vi "plant_structure.vi"(9 "Dataflow":errorcluster, 10 "Pause":refnum<vi>, 11 "Stop":refnum<vi>) -> ()   [LabVIEW 2019]
uses:
  lib/libSimulationControl/libSimulationControl.lvlib
panel:
  out "Dataflow Out":errorcluster
  # "*******************************************************************\nBiogas Plant Control\n\nAuthor: Paul Zügel\nGCSC-Frankfurt am Main 2020\n\n*******************************************************************"
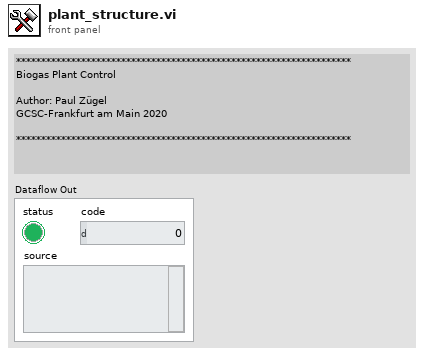
[diagram p1: front panel]
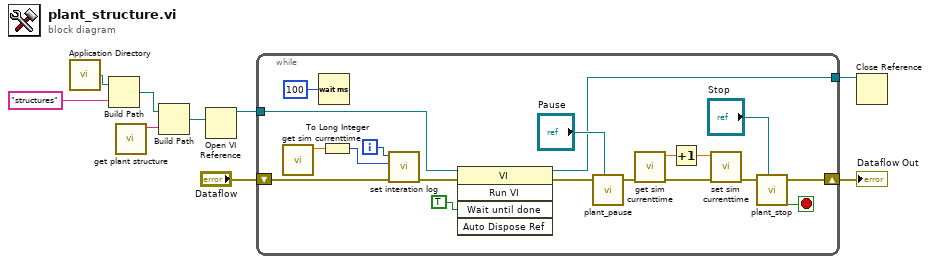
[diagram p0: block diagram]
diagram:
  n1 = call <vilib>:"Application Directory.vi"() -> ("Application Directory"=w7:path)
  n2 = Build Path(base path=w7, name or relative path="structures") -> (appended path=w5:path)
  n3 = call "get plant structure.vi"() -> ("function return"=w4:string)  [unwired: 10 in, 1 out]
  n4 = Build Path(base path=w5, name or relative path=w4) -> (appended path=w6:path)
  n5 = Open VI Reference(vi path=w6) -> (vi reference=w2:refnum<vi>)  [unwired: 5 in, 1 out]
  n6 = while {
    shift-right: [w25] -> w8
    shift-left: "Dataflow" -> [w15]
    tunnel: w2 -> [w13]
    tunnel: [w12] -> w1
    i -> [w24]
    stop <- w21 stop-if-true
    n7 = call "get sim currenttime.vi"() -> ("current_time"=w11:dbl)  [unwired: 10 in, 1 out]
    n8 = Wait (ms)(milliseconds to wait=u32 100) -> ()  [unwired: 1 out]
    n9 = To Long Integer(number=w11) -> (32bit integer=w10:i32)
    n10 = call "set interation log.vi"("error in (no error)"=w15, "time"=w10, "iter"=w24) -> ("error out"=w14:errorcluster)  [unwired: 8 in]
    n11 = invoke class="VI" method="Run VI"(reference=w13, error in=w14, "Wait until done"=TRUE ("Wait Until Done")) -> (reference out=w12:refnum<vi>, error out=w23:errorcluster)  [unwired: 2 in, 3 out]
    n12 = call "plant_pause.vi"("Dataflow In"=w23, "Pause"="Pause") -> ("Dataflow Out"=w18:errorcluster)  [unwired: 5 in]
    n13 = call "get sim currenttime.vi"("error in (no error)"=w18) -> ("error out"=w20:errorcluster, "current_time"=w16:dbl)  [unwired: 9 in]
    n14 = Increment(x=w16) -> (x+1=w19:dbl)
    n15 = call "set sim currenttime.vi"("error in (no error)"=w20, "time"=w19) -> ("error out"=w17:errorcluster)  [unwired: 9 in]
    n16 = call "plant_stop.vi"("Dataflow In"=w17, "Stop In"="Stop") -> ("Stop Out"=w21:bool, "Dataflow Out"=w25:errorcluster)  [unwired: 4 in]
  }
  "Dataflow Out" <- w8
  n17 = Close Reference(reference=w1) -> ()  [unwired: 1 in, 1 out]
